vi "Zmienna Globalna 02.vi"() -> ()   [LabVIEW 2020]
uses:
  Zmienna Globalna.vi
panel:
  in  "Szybkosc":i32
  in  "stop":bool
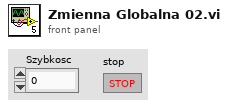
[diagram p1: front panel]
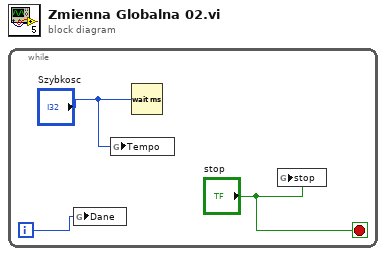
[diagram p0: block diagram]
diagram:
  n1 = while {
    i -> [w2]
    stop <- "stop" stop-if-true
    n2 = global write "Zmienna Globalna.vi" "Dane"(w2) -> ()
    n3 = global write "Zmienna Globalna.vi" "Tempo"("Szybkosc") -> ()
    n4 = Wait (ms)(milliseconds to wait="Szybkosc") -> ()  [unwired: 1 out]
    n5 = global write "Zmienna Globalna.vi" "stop"("stop") -> ()
  }
